vi "Run Child.vi"(8 "error in (no error)":errorcluster, 9 "Working Path":path, 10 "UI":refnum<class "UI.lvclass">, 11 "Build in":refnum<class "Build.lvclass">) -> (0 "error out":errorcluster, 3 "Build out":refnum<class "Build.lvclass">)   [LabVIEW 2020, in "Build.lvlib" / "Build.lvclass"]
uses:
  Build.lvclass
  build/ppl/neg-pkg.lvlibp/neg-pkg/UI/UI.lvclass
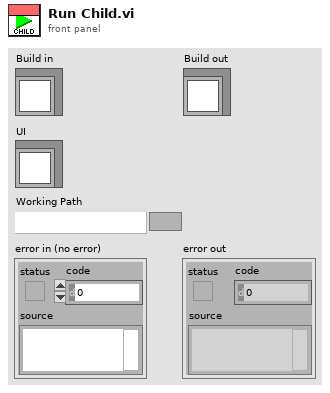
[diagram p1: front panel]
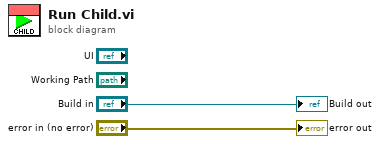
[diagram p0: block diagram]
diagram:
  "error out" <- "error in (no error)"
  "Build out" <- "Build in"
